vi "Close.vi"(8 "error in (no error)":errorcluster) -> (0 "error out":errorcluster)   [LabVIEW 2024, in "LogSingleton.lvlib"]
uses:
  LogSingleton.lvlib
  RQMHLogger/Logger.lvclass
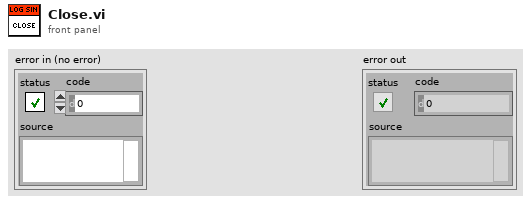
[diagram p1: front panel]
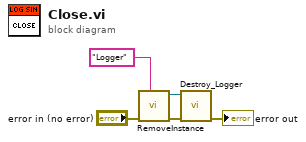
[diagram p0: block diagram]
diagram:
  n1 = call "RemoveInstance.vi"("Logger Name (Logger)"="Logger", "error in (no error)"="error in (no error)") -> ("error out"=w3:errorcluster, "RQMHLogger Get"=w2:refnum<class "Logger.lvclass">)  [unwired: 8 in]
  n2 = call "Destroy_Logger.vi"("error in (no error)"=w3, "RQMHLogger in"=w2) -> ("error out"=→"error out":errorcluster)  [unwired: 9 in]
